vi "read dependency small.vi"(8 "error in (no error)":errorcluster, 11 ".NET Refnum in":refnum<k24>) -> (0 "error out":errorcluster, 2 "Dependency":T1)   [LabVIEW 2015, in "Configuration Tool.lvlib"]
uses:
  Configuration Tool.lvlib
  NationalInstruments.VeriStand.XMLReader
  XML Controls/Dependency three item small.ctl
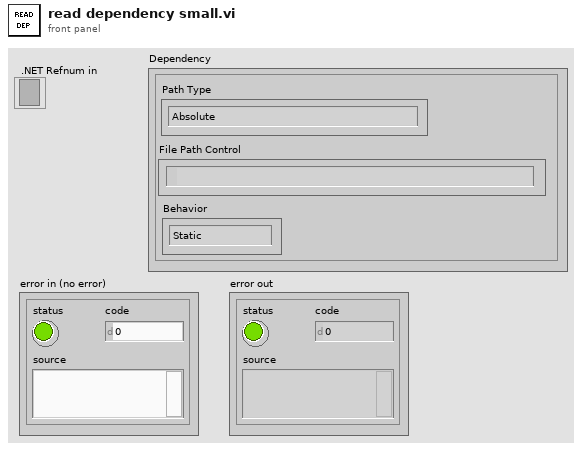
[diagram p1: front panel]
types:
  T1 = typedef "Configuration Tool.lvlib/Dependency three item small.ctl" = cluster{"File Path Control":path, "Path Type":enum16{"Absolute", "To Base", "To Common Doc Dir", "To Application Data Dir"}, "Behavior":enum16{"Static", "Dynamic"}}
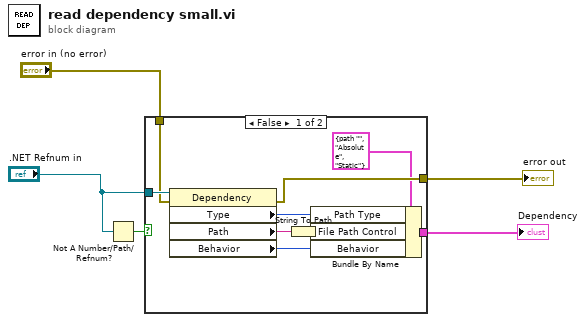
[diagram p0: block diagram]
diagram:
  n1 = Not A Number/Path/Refnum?(number/path/refnum=".NET Refnum in") -> (NaN/Path/Refnum?=w2:bool)
  n2 = case shown="False" w2 {
    tunnel: ".NET Refnum in" -> [w14 _]
    tunnel: [w11 _] -> w1
    tunnel: [w10 w15] -> w4
    tunnel: "error in (no error)" -> [w9 w15]
    frame False {
      n3 = property class="Dependency"(reference=w14, error in=w9) -> (error out=w10:errorcluster, "Type"=w7:i32, "Path"=w13:string, "Behavior"=w6:i32)  [unwired: 1 out]
      n4 = String To Path(string=w13) -> (path=w12:path)
      n5 = Bundle By Name(cluster=T1 {"File Path Control"=path "", "Path Type"=enum."Absolute", "Behavior"=enum."Static"} ("Dependency"), "Path Type"=w7, "File Path Control"=w12, "Behavior"=w6) -> (w11:T1)
    }
    frame True {
    }
  }
  "error out" <- w4
  "Dependency" <- w1
